vi "value array lv2.vi"(6 "Enum":T1, 7 "i":errorcluster, 8 "Value in":refnum<class "Value.lvclass">, 10 "serial":u32) -> (0 "out":errorcluster, 1 "out":refnum<class "Value.lvclass">, 2 "array out":refnum<class "Value.lvclass">[](array[class]))   [LabVIEW 2023, in "LabGRAD.lvlib" / "Value.lvclass"]
uses:
  Value.lvclass
  get set ini.ctl
  Value.lvclass/Value.ctl
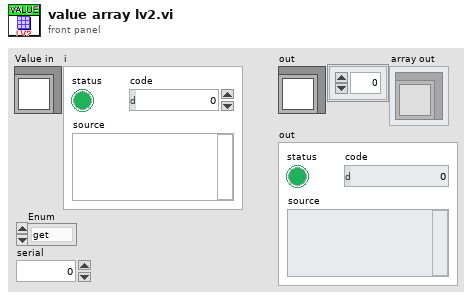
[diagram p1: front panel]
types:
  T1 = typedef "LabGRAD.lvlib/Value.lvclass/get set ini.ctl" = enum16{"get", "set", "ini"}
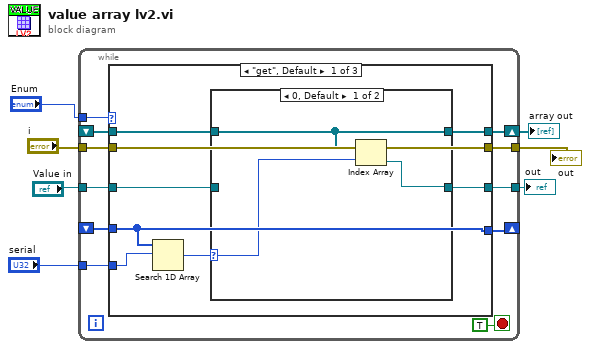
[diagram p0: block diagram]
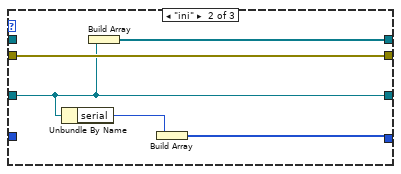
[diagram p3: hidden frame]
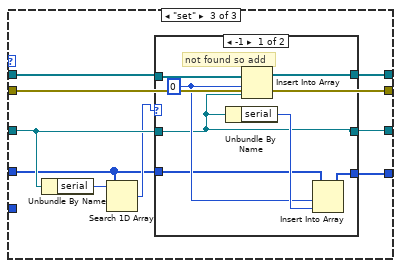
[diagram p4: hidden frame]
diagram:
  n1 = while {
    tunnel: "Enum" -> [w18]
    tunnel: "Value in" -> [w17]
    shift-right: [w16] -> w4
    shift-left: _ -> [w15]
    tunnel: "i" -> [w14]
    tunnel: [w13] -> w3
    tunnel: [w12] -> w5
    shift-right: [w10] -> _
    shift-left: _ -> [w9]
    tunnel: "serial" -> [w8]
    stop <- TRUE stop-if-true
    n2 = case shown="\"get\", Default" w18 {
      tunnel: w17 -> [w20 w34 w42]
      tunnel: [w21 w36 w43] -> w16
      tunnel: w15 -> [w22 _ w44]
      tunnel: w14 -> [w26 w35 w40]
      tunnel: [w26 w35 w40] -> w13
      tunnel: [w19 w34 w41] -> w12
      tunnel: [w25 w32 w39] -> w10
      tunnel: w9 -> [w25 _ w37]
      tunnel: w8 -> [w24 _ _]
      frame "get", Default {
        n3 = Search 1D Array(1D array=w25, element=w24) -> (index of element=w23:i32)  [unwired: 1 in]
        n4 = case shown="0, Default" w23 {
          selector: w23 -> [w28 _]
          tunnel: [w29 w31] -> w21
          tunnel: w22 -> [w29 w31]
          tunnel: w20 -> [_ w30]
          tunnel: [w27 w30] -> w19
          frame 0, Default {
            n5 = Index Array(array=w29, index=w28) -> (element=w27:refnum<class "Value.lvclass">)
          }
          frame -1 {
          }
        }
      }
      frame "ini" {
        n6 = Unbundle By Name(w34) -> ("serial"=w33:u32)
        n7 = Build Array(w34) -> (w36:refnum<class "Value.lvclass">[])
        n8 = Build Array(w33) -> (w32:u32[])
      }
      frame "set" {
        n9 = Unbundle By Name(w42) -> ("serial"=w45:u32)
        n10 = Search 1D Array(1D array=w37, element=w45) -> (index of element=w38:i32)  [unwired: 1 in]
        n11 = case shown="-1" w38 {
          tunnel: w44 -> [w52 w53]
          tunnel: [w51 w53] -> w43
          tunnel: w42 -> [w46 w55]
          tunnel: [w48 w54] -> w39
          tunnel: w37 -> [w47 w54]
          tunnel: [w46 w55] -> w41
          frame -1 {
            w49 = 0 ("index")
            # "not found so add"
            n12 = Unbundle By Name(w46) -> ("serial"=w50:u32)
            n13 = Insert Into Array(array=w52, index=w49, new element=w46) -> (w51:refnum<class "Value.lvclass">[])
            n14 = Insert Into Array(array=w47, index=w49, new element=w50) -> (w48:u32[])
          }
          frame 1, Default {
            # "already in array"
          }
        }
      }
    }
  }
  "out" <- w5
  "array out" <- w4
  "out" <- w3
